vi "NI VeriStand - Get Single Channel Value.vi"(8 "error in (no error)":errorcluster, 10 "Channel":string, 11 "WorkspaceManager in":T1) -> (0 "error out":errorcluster, 2 "Value":dbl, 3 "WorkspaceManager out":T1)   [LabVIEW 2020, in "NI_VS Workspace ExecutionAPI.lvlib"]
doc: "Returns values of channels on the target. You can get values for a single channel, multiple channels, or vector values for a single channel. You must manually select the polymorphic instance to use."
uses:
  <vilib>/NI VeriStand/Execution/Workspace/NI_VS Workspace ExecutionAPI.lvlib
  <vilib>/NI VeriStand/Execution/Workspace/WorkspaceAPI.ctl
  NationalInstruments.VeriStand.ClientAPI
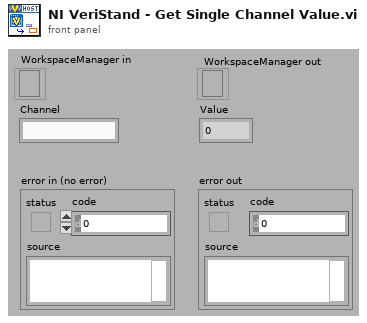
[diagram p1: front panel]
types:
  T1 = typedef "NI_VS Workspace ExecutionAPI.lvlib/WorkspaceAPI.ctl" = refnum<k24>
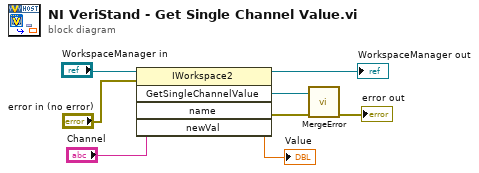
[diagram p0: block diagram]
diagram:
  n1 = invoke class="IWorkspace2" method="GetSingleChannelValue"(reference="WorkspaceManager in", error in="error in (no error)", "name"="Channel") -> (reference out=→"WorkspaceManager out":T1, error out=w6:errorcluster, "GetSingleChannelValue"=w5:refnum<k24>, "newVal"=→"Value":dbl)  [unwired: 2 in, 1 out]
  n2 = call <vilib>:"MergeError.vi"("error in (no error)"=w6, "Error"=w5) -> ("error out"=→"error out":errorcluster)  [unwired: 9 out]
